vi "CreateNew_GetCreateNewWeight.vi"() -> ()   [LabVIEW 2020, in "FlexWorker_Provider.lvlib"]
uses:
  FlexWorker_Provider.lvlib
  <resource>/Framework/Providers/API/ItemRef.ctl
panel:
  out "Weight":i32
  in  "Wizard":T1
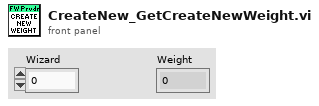
[diagram p1: front panel]
types:
  T1 = typedef "ItemRef.ctl" = u64
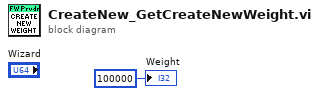
[diagram p0: block diagram]
diagram:
  "Weight" <- 100000 ("Weight")
